vi "ATMonochromator_getEvent_settingsAppliedMonoCommunication.vi"(8 "error in (no error)":errorcluster, 11 "logevent_settingsAppliedMonoCommunication_Ctl":T1) -> (0 "error out":errorcluster, 2 "function return":i32, 3 "logevent_settingsAppliedMonoCommunication_Ctl out":T1)   [LabVIEW 2016, in "SALLV_ATMonochromator.lvlib"]
doc: "int ATMonochromator_shm_getEvent_settingsAppliedMonoCommunicationLV(ATMonochromator_logevent_settingsAppliedMonoCommunicationLV *logevent_settingsAppliedMonoCommunication_Ctl );"
uses:
  SALLV_ATMonochromator.lvlib
  DataTypes/logevent_settingsAppliedMonoCommunication.ctl
  SALLV_ATMonochromator.so
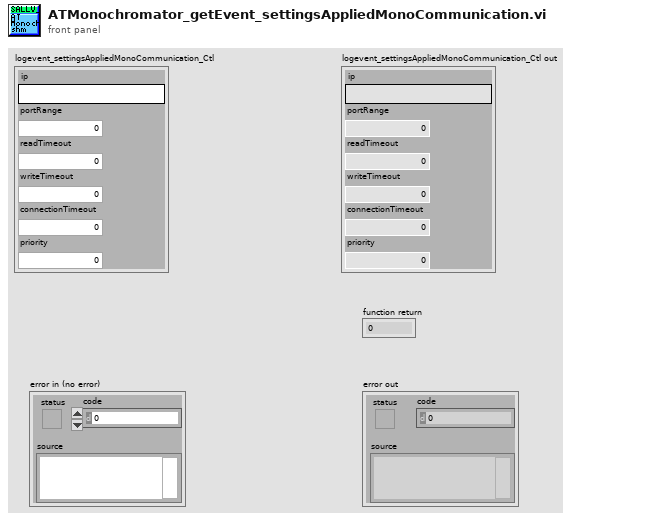
[diagram p1: front panel]
types:
  T1 = typedef "SALLV_ATMonochromator.lvlib/logevent_settingsAppliedMonoCommunication.ctl" = cluster{"ip":string, "portRange":i32, "readTimeout":sgl, "writeTimeout":sgl, "connectionTimeout":sgl, "priority":i32}
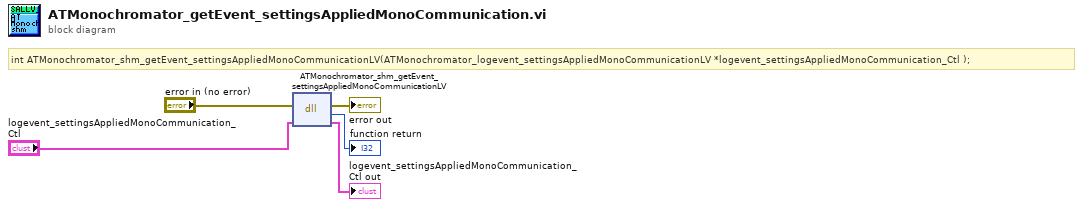
[diagram p0: block diagram]
diagram:
  # "int ATMonochromator_shm_getEvent_settingsAppliedMonoCommunicationLV(ATMonochromator_logevent_settingsAppliedMonoCommunicationLV *logevent_settingsAppliedMonoCommunication_Ctl );"
  n1 = dll-call lib="home/harini/tcs/SALLV_ATMonochromator/SALLV_ATMonochromator.*" fn="ATMonochromator_shm_getEvent_settingsAppliedMonoCommunicationLV"(error in="error in (no error)", "logevent_settingsAppliedMonoCommunication_Ctl"="logevent_settingsAppliedMonoCommunication_Ctl") -> (error out=→"error out":errorcluster, →"function return":i32, "logevent_settingsAppliedMonoCommunication_Ctl"=→"logevent_settingsAppliedMonoCommunication_Ctl out":T1)  [unwired: 2 in, 1 out]
